vi "EventLog.Gui.Run.vi"(8 "error in":errorcluster) -> (0 "error out":errorcluster, 3 "Ref":refnum<vi>)   [LabVIEW 2016]
uses:
  Tma.lib/string.llb/Join array to string.vi
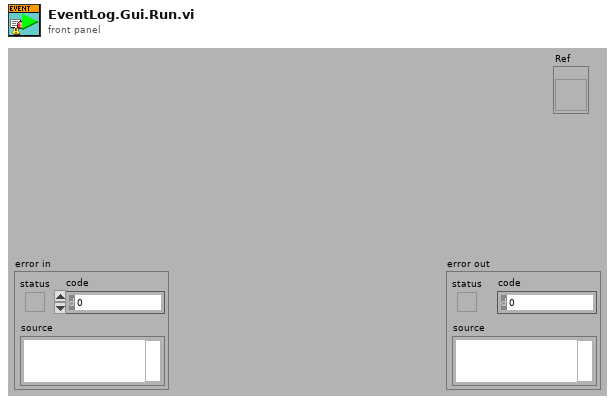
[diagram p1: front panel]
types:
  T1 = enum32{"Bad", "Idle", "Run top level", "Running"}
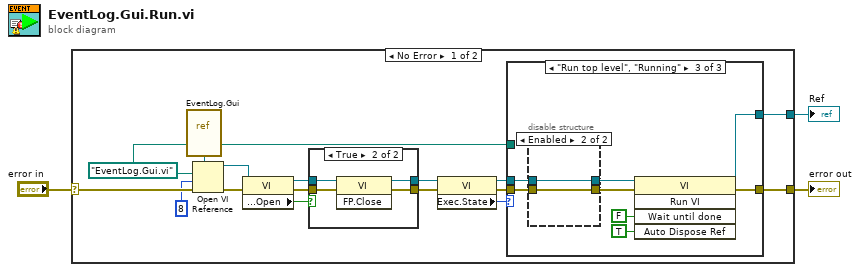
[diagram p0: block diagram]
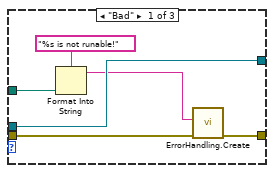
[diagram p3: hidden frame]
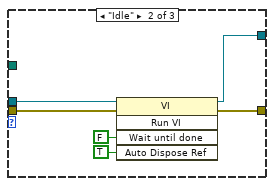
[diagram p4: hidden frame]
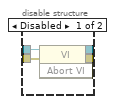
[diagram p5: hidden frame]
diagram:
  n1 = case shown="No Error" "error in" {
    selector: "error in" -> [w17 w52]
    tunnel: [w13 w52] -> w3
    tunnel: [w14 _] -> w1
    frame No Error {
      w4 = path "EventLog.Gui.vi" ("vi path")
      n2 = vi-ref "EventLog.Gui.vi"() -> (w18:refnum<vi>)
      n3 = Open VI Reference(type specifier VI Refnum (for type only)=w18, vi path=w4, options=8, error in (no error)=w17) -> (vi reference=w8:refnum<vi>, error out=w9:errorcluster)  [unwired: 2 in]
      n4 = property class="VI"(reference=w8, error in=w9) -> (reference out=w10:refnum<vi>, error out=w12:errorcluster, "Front Panel.Open"=w11:bool)
      n5 = case shown="True" w11 {
        tunnel: [w20 w25] -> w6
        tunnel: [w21 w24] -> w7
        tunnel: w12 -> [w20 w23]
        tunnel: w10 -> [w21 w22]
        frame False {
        }
        frame True {
          n6 = invoke class="VI" method="FP.Close"(reference=w22, error in=w23) -> (reference out=w24:refnum<vi>, error out=w25:errorcluster)  [unwired: 1 in, 1 out]
        }
      }
      n7 = property class="VI"(reference=w7, error in=w6) -> (reference out=w15:refnum<vi>, error out=w16:errorcluster, "Exec.State"=w19:T1)
      n8 = case shown="\"Run top level\", \"Running\"" w19 {
        tunnel: [w29 w36 w39] -> w13
        tunnel: w16 -> [w30 w34 w40]
        tunnel: [w31 w35 w38] -> w14
        tunnel: w15 -> [w31 w37 w41]
        tunnel: w4 -> [w28 _ _]
        frame "Bad" {
          n9 = Format Into String(format string="%s is not runable!" ("explanation"), w28) -> (resulting string=w26:string)  [unwired: 2 in, 1 out]
          n10 = call "ErrorHandling.Create.vi"("error in"=w30, "explanation"=w26) -> ("error out"=w29:errorcluster)  [unwired: 9 in]
        }
        frame "Idle" {
          n11 = invoke class="VI" method="Run VI"(reference=w37, error in=w34, "Wait until done"=FALSE ("Wait Until Done"), "Auto Dispose Ref"=TRUE ("Auto Dispose Reference")) -> (reference out=w35:refnum<vi>, error out=w36:errorcluster)  [unwired: 1 in, 3 out]
        }
        frame "Run top level", "Running" {
          n12 = disable-structure shown="Enabled" {
            disable-tunnel: [w49 w51] -> w43
            disable-tunnel: [w48 w50] -> w42
            disable-tunnel: w41 -> [w47 w50]
            disable-tunnel: w40 -> [w46 w51]
            frame Disabled {
              n13 = invoke class="VI" method="Abort VI"(reference=w47, error in=w46) -> (reference out=w48:refnum<vi>, error out=w49:errorcluster)  [unwired: 1 in, 1 out]
            }
            frame Enabled {
            }
          }
          n14 = invoke class="VI" method="Run VI"(reference=w42, error in=w43, "Wait until done"=FALSE ("Wait Until Done"), "Auto Dispose Ref"=TRUE ("Auto Dispose Reference")) -> (reference out=w38:refnum<vi>, error out=w39:errorcluster)  [unwired: 1 in, 3 out]
        }
      }
    }
    frame Error {
    }
  }
  "error out" <- w3
  "Ref" <- w1
